vi "write_log_metadata.vi"(8 "error in (no error)":errorcluster, 10 "data":variant, 11 "scan_hdf5_log in":refnum<class "scan_hdf5_log.lvclass">) -> (0 "error out":errorcluster, 3 "scan_hdf5_log out":refnum<class "scan_hdf5_log.lvclass">)   [LabVIEW 2015, in "scan_hdf5_log.lvclass"]
uses:
  scan_hdf5_log.lvclass
  scan_settings.ctl
  scan_unit.ctl
  scan_record.ctl
  scan_hdf5_log.lvclass/scan_hdf5_log.ctl
  <vilib>/UPVI/lvhdf5/attribute.llb/Simple H5Awrite (Variant).vi
  <vilib>/UPVI/lvhdf5/attribute.llb/LVH5A Operation.ctl
  <vilib>/UPVI/lvhdf5/attribute.llb/Simple H5Awrite.xnode
  <vilib>/UPVI/lvhdf5/library.llb/HDF5 Ref.ctl
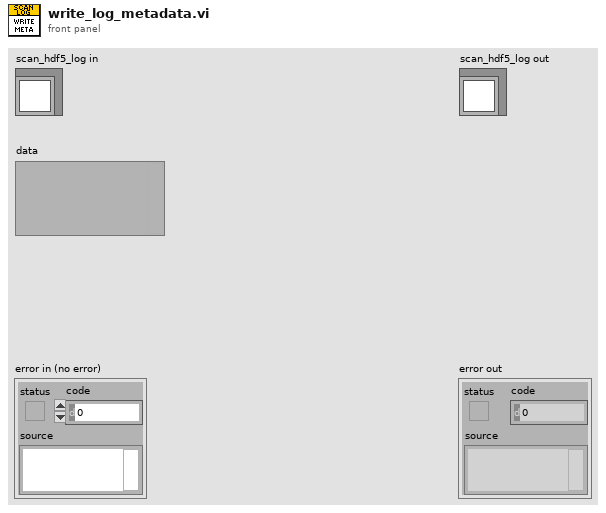
[diagram p1: front panel]
types:
  T1 = typedef "scan_settings.ctl" = cluster{"Center Pos. (mm)":dbl, "Range [--|--]":dbl, "Unit":T2, "Steps":dbl, "Stage Number":enum16{"1", "2"}, "Stage Speed":dbl, "Dwell Time (s)":dbl, "Record Type":T3, "Save Path":path, "Notes":string}
  T2 = typedef "scan_unit.ctl" = enum16{"mm", "s", "ms", "us", "ns", "ps", "fs"}
  T3 = typedef "scan_record.ctl" = enum16{"hdf5", "legacy", "None"}
  T4 = typedef "LVH5A Operation.ctl" = enum16{"open", "replace", "create", "open or create", "create or replace", "create or replace with confirmation"}
  T5 = typedef "HDF5 Ref.ctl" = refnum<k1>
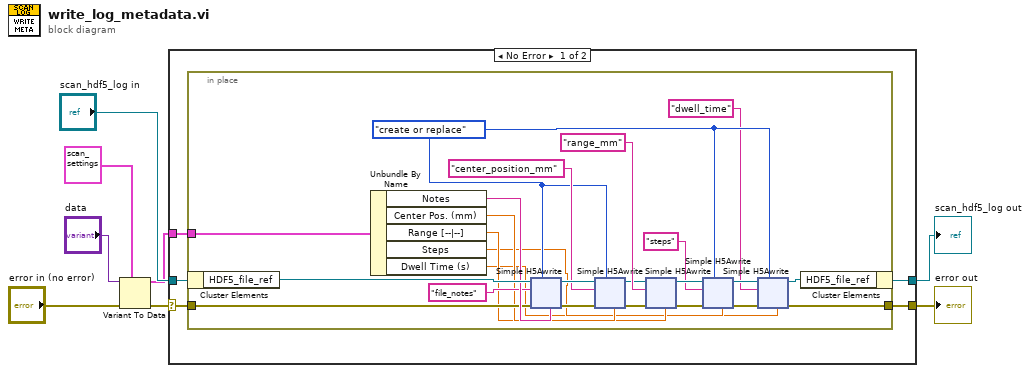
[diagram p0: block diagram]
diagram:
  n1 = Variant To Data(error in="error in (no error)", type=T1 {"Center Pos. (mm)"=0.0, "Range [--|--]"=0.0, "Unit"=enum."mm", "Steps"=0.0, "Stage Number"=enum."1", "Stage Speed"=1.0, "Dwell Time (s)"=0.1, "Record Type"=enum."hdf5", "Save Path"=path "", "Notes"=""} ("scan_settings"), Variant="data") -> (data=w3:T1, error out=w5:errorcluster)
  n2 = case shown="No Error" w5 {
    selector: w5 -> [w11 w113]
    tunnel: "scan_hdf5_log in" -> [w13 w114]
    tunnel: w3 -> [w12 _]
    tunnel: [w10 w113] -> w2
    tunnel: [w9 w114] -> w1
    frame No Error {
      n3 = in-place {
        in-place-border: w12 -> [w36]
        in-place-border: w11 -> [w33]
        in-place-border: [w14] -> w10
        w20 = LVH5A_Operation."create or replace" ("operation (open or create)")
        n4 = in-place-cluster #1(w13) -> ("HDF5_file_ref"=w37:T5)
        n5 = Unbundle By Name(w36) -> ("Notes"=w35:string, "Center Pos. (mm)"=w29:dbl, "Range [--|--]"=w27:dbl, "Steps"=w18:dbl, "Dwell Time (s)"=w17:dbl)
        n6 = xnode "Simple H5Awrite"("HDF5 Ref"=w37, "Name"="file_notes", "error in (no error)"=w33, "operation (open or create)"=w20, "Value"=w35) -> ("HDF5 Ref out"=w31:T5, "error out"=w32:errorcluster)
        n7 = xnode "Simple H5Awrite"("HDF5 Ref"=w31, "Name"="center_position_mm", "error in (no error)"=w32, "operation (open or create)"=w20, "Value"=w29) -> ("HDF5 Ref out"=w23:T5, "error out"=w28:errorcluster)
        n8 = xnode "Simple H5Awrite"("HDF5 Ref"=w23, "Name"="range_mm", "error in (no error)"=w28, "Value"=w27) -> ("HDF5 Ref out"=w25:T5, "error out"=w24:errorcluster)  [unwired: 1 in]
        n9 = xnode "Simple H5Awrite"("HDF5 Ref"=w25, "Name"="steps", "error in (no error)"=w24, "operation (open or create)"=w20, "Value"=w18) -> ("HDF5 Ref out"=w22:T5, "error out"=w21:errorcluster)
        n10 = xnode "Simple H5Awrite"("HDF5 Ref"=w22, "Name"="dwell_time", "error in (no error)"=w21, "operation (open or create)"=w20, "Value"=w17) -> ("HDF5 Ref out"=w15:T5, "error out"=w14:errorcluster)
        n11 = in-place-cluster #1("HDF5_file_ref"=w15) -> (w9:refnum<class "scan_hdf5_log.lvclass">)
      }
    }
    frame Error {
    }
  }
  "error out" <- w2
  "scan_hdf5_log out" <- w1
